vi "Display Waveform.vi"() -> ()   [LabVIEW 2018]
panel:
  in  "stop":bool
  out "Waveform Chart":dbl(graph)
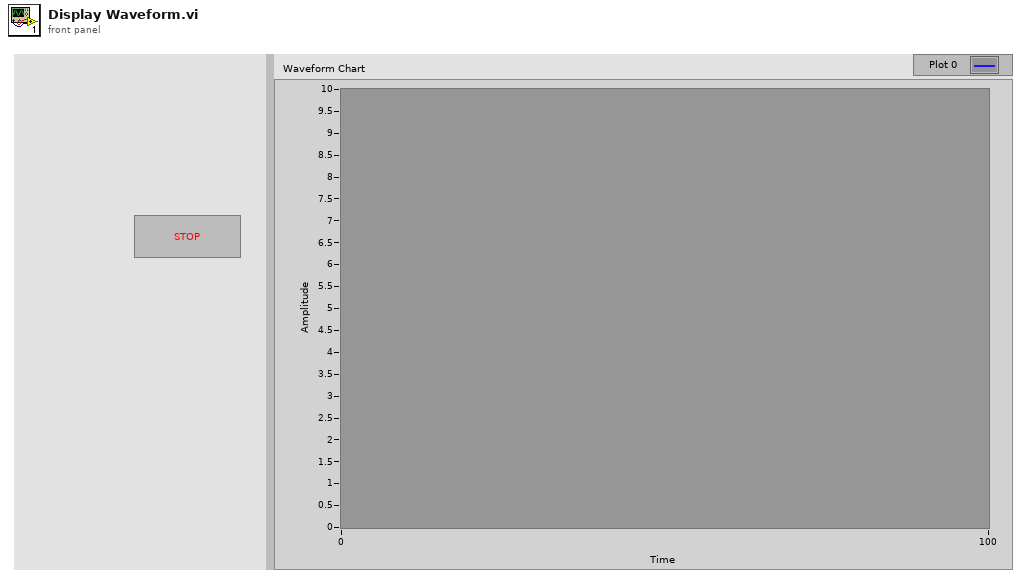
[diagram p1: front panel]
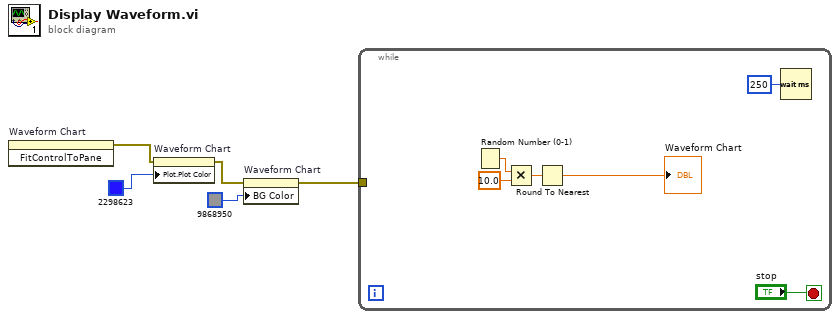
[diagram p0: block diagram]
diagram:
  n1 = invoke on="Waveform Chart" class="WFChart (strict)" method="FitControlToPane"() -> (error out=w1:errorcluster)  [unwired: 3 in, 2 out]
  n2 = property on="Waveform Chart" class="WFChart (strict)"(error in=w1, "Plot.Plot Color"=u32 2298623) -> (error out=w4:errorcluster)  [unwired: 1 in, 1 out]
  n3 = property on="Waveform Chart" class="WFChart (strict)"(error in=w4, "BG Color"=u32 9868950) -> (error out=w3:errorcluster)  [unwired: 1 in, 1 out]
  n4 = while {
    tunnel: w3 -> [_]
    stop <- "stop" stop-if-true
    n5 = Random Number (0-1)() -> (number: 0 to 1=w9:dbl)
    n6 = Multiply(x=w9, y=10.0) -> (x*y=w7:dbl)
    n7 = Round To Nearest(number=w7) -> (nearest integer value=→"Waveform Chart":dbl)
    n8 = Wait (ms)(milliseconds to wait=u32 250) -> ()  [unwired: 1 out]
  }
